vi "Remove Autogrow from Structures.vi"(8 "error in (no error)":errorcluster, 11 "vi path":path) -> (0 "error out":errorcluster)   [LabVIEW 2020]
uses:
  <vilib>/Utility/traverseref.llb/TRef TravTarget.ctl
  <vilib>/Utility/traverseref.llb/VI Scripting - Traverse.lvlib
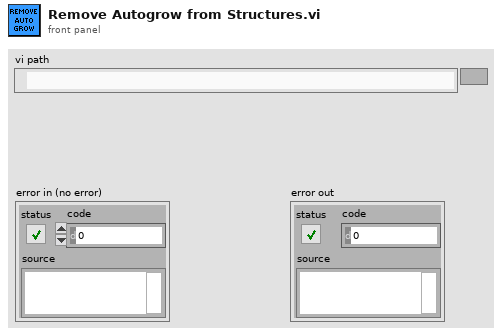
[diagram p1: front panel]
types:
  T1 = typedef "TRef TravTarget.ctl" = enum16{"FP", "BD", "Other"}
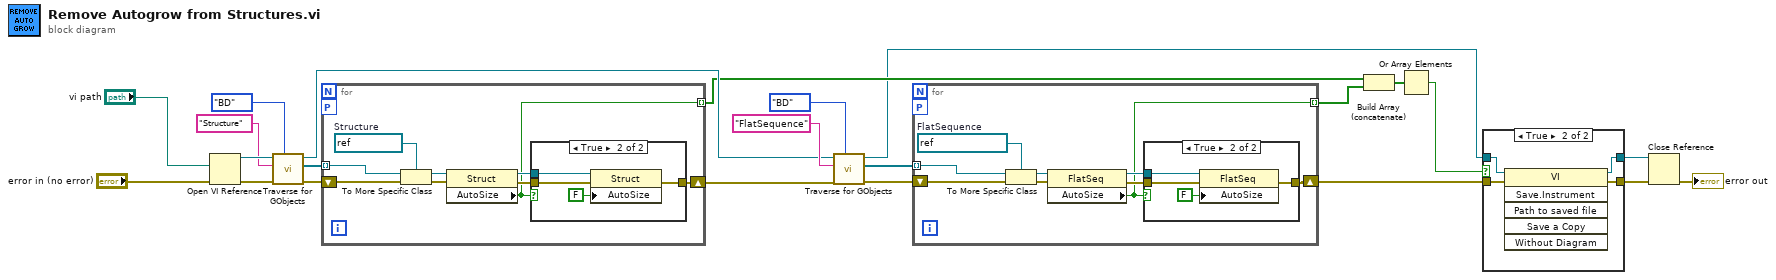
[diagram p0: block diagram]
diagram:
  n1 = Open VI Reference(vi path="vi path", error in (no error)="error in (no error)") -> (vi reference=w17:refnum<vi>, error out=w18:errorcluster)  [unwired: 4 in]
  n2 = call <vilib>:"Traverse for GObjects.vi"("Traverse Target"=TRef_TravTarget."BD", "error in (no error)"=w18, "Class Name"="Structure", "VI Refnum"=w17) -> ("error out"=w15:errorcluster, "References"=w14:refnum<vi>[], "dup VI Refnum"=w11:refnum<vi>)  [unwired: 4 in, 1 out]
  n3 = for {
    tunnel: w14 -> [w32] mode=indexing
    tunnel: [w25] -> w6 mode=indexing
    shift-right: [w24] -> w12
    shift-left: w15 -> [w26]
    workers-P: _ -> [_]
    w31 = refnum<vi> refnum  # Structure
    n4 = To More Specific Class(target class=w31, reference=w32, error in=w26) -> (specific class reference=w30:refnum<vi>, error out=w28:errorcluster)
    n5 = property class="Struct"(reference=w30, error in=w28) -> (reference out=w29:refnum<vi>, error out=w27:errorcluster, "AutoSize"=w25:bool)
    n6 = case shown="True" w25 {
      tunnel: w29 -> [_ w37]
      tunnel: w27 -> [w33 w36]
      tunnel: [w33 w34] -> w24
      frame False {
      }
      frame True {
        n7 = property class="Struct"(reference=w37, error in=w36, "AutoSize"=FALSE ("AutoSize To Fit Contents?")) -> (error out=w34:errorcluster)  [unwired: 1 out]
      }
    }
  }
  n8 = call <vilib>:"Traverse for GObjects.vi"("Traverse Target"=TRef_TravTarget."BD", "error in (no error)"=w12, "Class Name"="FlatSequence", "VI Refnum"=w11) -> ("error out"=w10:errorcluster, "References"=w9:refnum<vi>[], "dup VI Refnum"=w4:refnum<vi>)  [unwired: 4 in, 1 out]
  n9 = for {
    tunnel: w9 -> [w46] mode=indexing
    tunnel: [w39] -> w7 mode=indexing
    shift-right: [w38] -> w8
    shift-left: w10 -> [w40]
    workers-P: _ -> [_]
    w45 = refnum<vi> refnum  # FlatSequence
    n10 = To More Specific Class(target class=w45, reference=w46, error in=w40) -> (specific class reference=w44:refnum<vi>, error out=w42:errorcluster)
    n11 = property class="FlatSeq"(reference=w44, error in=w42) -> (reference out=w43:refnum<vi>, error out=w41:errorcluster, "AutoSize"=w39:bool)
    n12 = case shown="True" w39 {
      tunnel: w43 -> [_ w51]
      tunnel: w41 -> [w47 w50]
      tunnel: [w47 w48] -> w38
      frame False {
      }
      frame True {
        n13 = property class="FlatSeq"(reference=w51, error in=w50, "AutoSize"=FALSE ("AutoSize To Fit Contents?")) -> (error out=w48:errorcluster)  [unwired: 1 out]
      }
    }
  }
  n14 = Build Array (concatenate)(w6, w7) -> (w5:bool[])
  n15 = Or Array Elements(Boolean array=w5) -> (logical OR=w3:bool)
  n16 = case shown="True" w3 {
    tunnel: w8 -> [w53 w57]
    tunnel: [w53 w56] -> w20
    tunnel: [w52 w55] -> w19
    tunnel: w4 -> [w52 w54]
    frame False {
    }
    frame True {
      n17 = invoke class="VI" method="Save.Instrument"(reference=w54, error in=w57) -> (reference out=w55:refnum<vi>, error out=w56:errorcluster)  [unwired: 4 in, 4 out]
    }
  }
  n18 = Close Reference(reference=w19, error in (no error)=w20) -> (error out=→"error out":errorcluster)
